vi "Poisson Inverse CDF.vi"(10 "lambda":dbl=1.0, 11 "cdf(x)":dbl) -> (0 "error":i32, 3 "x":i32)   [LabVIEW 2018, in "NI_Gmath.lvlib"]
doc: "Computes the discrete inverse cumulative distribution function (CDF), or the value <B>x</B> such that the probability that the random variate X, where X describes the selected distribution type, takes on a value less than or equal to it is <B>cdf(x)</B>. You must manually select the polymorphic instance to use."
uses:
  NI_Gmath.lvlib
panel:
  # "Poisson Inverse CDF"
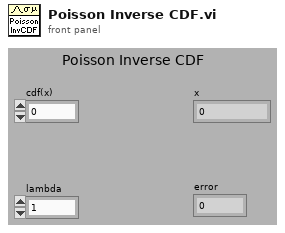
[diagram p1: front panel]
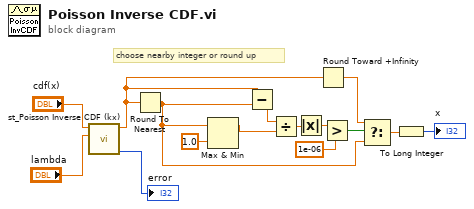
[diagram p0: block diagram]
diagram:
  # "choose nearby integer or round up"
  n1 = call "st_Poisson Inverse CDF (kx).vi"("lambda"="lambda", "cdf(x)"="cdf(x)") -> ("error"=→"error":i32, "x"=w6:dbl)  [unwired: 8 in]
  n2 = Round To Nearest(number=w6) -> (nearest integer value=w2:dbl)
  n3 = Max & Min(x=w2, y=1.0) -> (max(x,y)=w1:dbl)  [unwired: 1 out]
  n4 = Subtract(x=w6, y=w2) -> (x-y=w14:dbl)
  n5 = Divide(x=w14, y=w1) -> (x/y=w12:dbl)
  n6 = Absolute Value(x=w12) -> (abs(x)=w13:dbl)
  n7 = Round Toward +Infinity(x=w6) -> (ceil(x): smallest int >= x=w9:dbl)
  n8 = Greater?(x=w13, y=1e-06) -> (0:w10:bool)
  n9 = Select(t=w9, s=w10, f=w2) -> (s? t:f=w15:dbl)
  n10 = To Long Integer(number=w15) -> (32bit integer=→"x":i32)
